vi "Stop Test.vi"(8 "error in (no error)":errorcluster, 11 "Coverage Analyzer in":refnum<class "Coverage Analyzer.lvclass">) -> (0 "error out":errorcluster, 3 "Coverage Analyzer out":refnum<class "Coverage Analyzer.lvclass">)   [LabVIEW 2020, in "Coverage Analyzer.lvlib" / "Coverage Analyzer.lvclass"]
uses:
  Coverage Analyzer.lvclass
  Coverage Analyzer.lvclass/Coverage Analyzer.ctl
  Private/Coverage Analyzer View.vi
  b1335121-492a-44c3-aab0-280f61647e09.vi
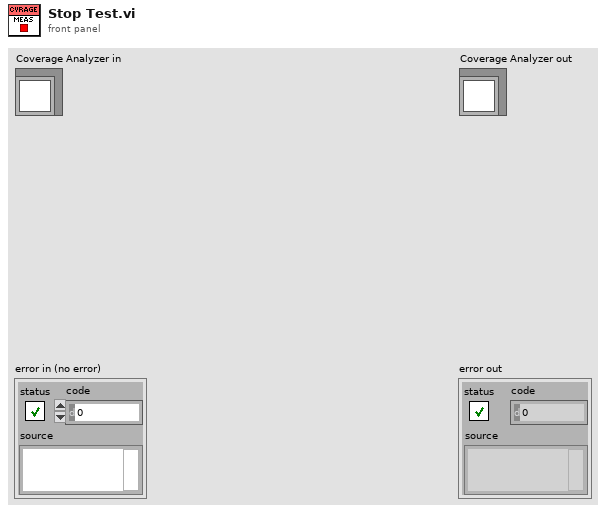
[diagram p1: front panel]
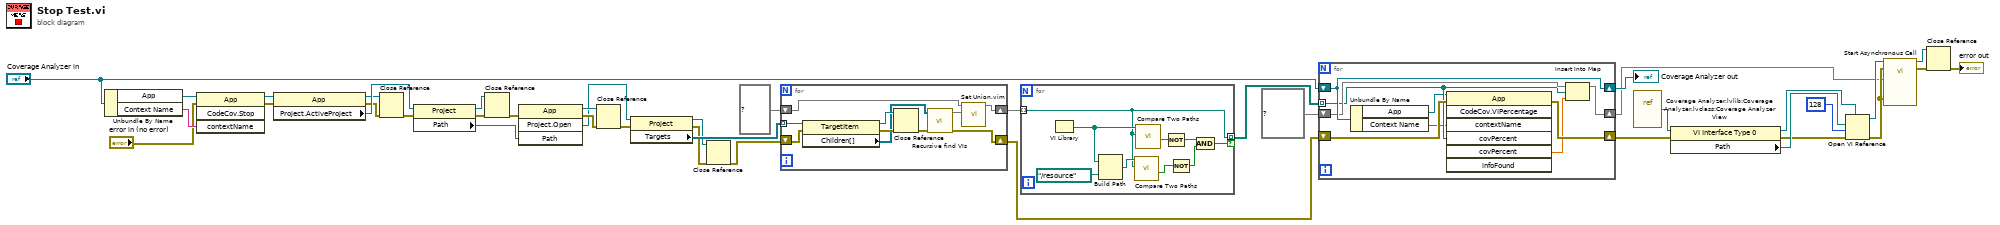
[diagram p0: block diagram]
diagram:
  n1 = Unbundle By Name("Coverage Analyzer in") -> ("App"=w40:refnum<vi>, "Context Name"=w39:string)
  n2 = invoke class="App" method="CodeCov.Stop"(reference=w40, error in="error in (no error)", "contextName"=w39) -> (reference out=w31:refnum<vi>, error out=w16:errorcluster)  [unwired: 1 in, 2 out]
  n3 = property class="App"(reference=w31, error in=w16) -> (reference out=w36:refnum<vi>, error out=w33:errorcluster, "Project.ActiveProject"=w37:refnum<vi>)
  n4 = Close Reference(reference=w36, error in (no error)=w33) -> (error out=w32:errorcluster)
  n5 = property class="Project"(reference=w37, error in=w32) -> (reference out=w35:refnum<vi>, error out=w34:errorcluster, "Path"=w19:path)
  n6 = Close Reference(reference=w35, error in (no error)=w34) -> (error out=w15:errorcluster)
  n7 = invoke class="App" method="Project.Open"(error in=w15, "Path"=w19) -> (reference out=w9:refnum<vi>, error out=w5:errorcluster, "Project:Open"=w3:refnum<vi>)  [unwired: 2 in, 1 out]
  n8 = Close Reference(reference=w9, error in (no error)=w5) -> (error out=w8:errorcluster)
  n9 = property class="Project"(reference=w3, error in=w8) -> (reference out=w7:refnum<vi>, error out=w4:errorcluster, "Targets"=w12:refnum<vi>[])
  n10 = Close Reference(reference=w7, error in (no error)=w4) -> (error out=w6:errorcluster)
  n11 = for {
    tunnel: w12 -> [w50] mode=indexing
    shift-right: [w47] -> w21
    shift-left: w6 -> [w48]
    shift-right: [w43] -> w11
    shift-left: set{path} {} ("VIs") -> [w45]
    n12 = property class="TargetItem"(reference=w50, error in=w48) -> (reference out=w46:refnum<vi>, error out=w49:errorcluster, "Children[]"=w41:refnum<vi>[])
    n13 = Close Reference(reference=w46, error in (no error)=w49) -> (error out=w42:errorcluster)
    n14 = call "Recursive find VIs.vi"("error in (no error)"=w42, "Project Items"=w41) -> ("error out"=w47:errorcluster, "VIs"=w44:set{path})  [unwired: 8 in]
    n15 = call "Set Union.vim"("set 2"=w44, "set 1"=w45) -> ("union"=w43:set{path})  [unwired: 9 in]
  }
  n16 = for {
    tunnel: w11 -> [w51] mode=indexing
    tunnel: [w51] -> w1 mode=indexing if=w56
    n17 = VI Library() -> (path=w54:path)
    n18 = Build Path(base path=w54, name or relative path=path "../resource") -> (appended path=w52:path)
    n19 = call <vilib>:"Compare Two Paths.vi"("Path 2"=w51, "Path 1"=w52) -> ("Path 2 Relative to Path 1?"=w57:bool)  [unwired: 6 in, 3 out]
    n20 = call <vilib>:"Compare Two Paths.vi"("Path 2"=w51, "Path 1"=w54) -> ("Path 2 Relative to Path 1?"=w59:bool)  [unwired: 6 in, 3 out]
    n21 = Not(x=w59) -> (.not. x?=w58:bool)
    n22 = Not(x=w57) -> (.not. x?=w55:bool)
    n23 = And(x=w58, y=w55) -> (x .and. y?=w56:bool)
  }
  n24 = for {
    shift-right: [w68] -> w17
    shift-left: "Coverage Analyzer in" -> [w68]
    shift-right: [w66] -> w20
    shift-left: w21 -> [w67]
    tunnel: w1 -> [w63] mode=indexing
    shift-right: [w64] -> w2
    shift-left: map{path, dbl} {} ("Code Coverage") -> [w65]
    n25 = Unbundle By Name(w68) -> ("App"=w60:refnum<vi>, "Context Name"=w61:string)
    n26 = invoke class="App" method="CodeCov.VIPercentage"(reference=w60, error in=w67, "contextName"=w61, "covPercent"=w63) -> (error out=w66:errorcluster, "covPercent"=w62:dbl)  [unwired: 3 in, 5 out]
    n27 = Insert Into Map(map in=w65, key=w63, value=w62) -> (map out=w64:map{path, dbl})  [unwired: 2 out]
  }
  "Coverage Analyzer out" <- w17
  n28 = vi-ref "Coverage Analyzer.lvlib:Coverage Analyzer.lvclass:Coverage Analyzer View.vi"() -> (w23:refnum<vi>)
  n29 = property class="VI Interface Type 0"(reference=w23, error in=w20) -> (reference out=w27:refnum<vi>, error out=w25:errorcluster, "Path"=w26:path)
  n30 = Open VI Reference(type specifier VI Refnum (for type only)=w27, vi path=w26, options=128, error in (no error)=w25) -> (vi reference=w22:refnum<vi>, error out=w24:errorcluster)  [unwired: 2 in]
  n31 = call-by-ref "Start Asynchronous Call"(reference=w22, error in=w24, 8:"error in (no error)"=w24, "Code Coverage"=w2) -> (reference out=w30:refnum<vi>, error out=w29:errorcluster)  [unwired: 9 in, 1 out]
  n32 = Close Reference(reference=w30, error in (no error)=w29) -> (error out=→"error out":errorcluster)
